vi "SHA-2_hash chunk_U64.vi"(0 "h in":u64[](array[numeric]), 1 "Chunk":u64[](array[numeric]), 12 "error in (no error)":errorcluster) -> (4 "h out":u64[](array[numeric]), 14 "error out":errorcluster)   [LabVIEW 2012, in "Encryption.lvlib"]
uses:
  Encryption.lvlib
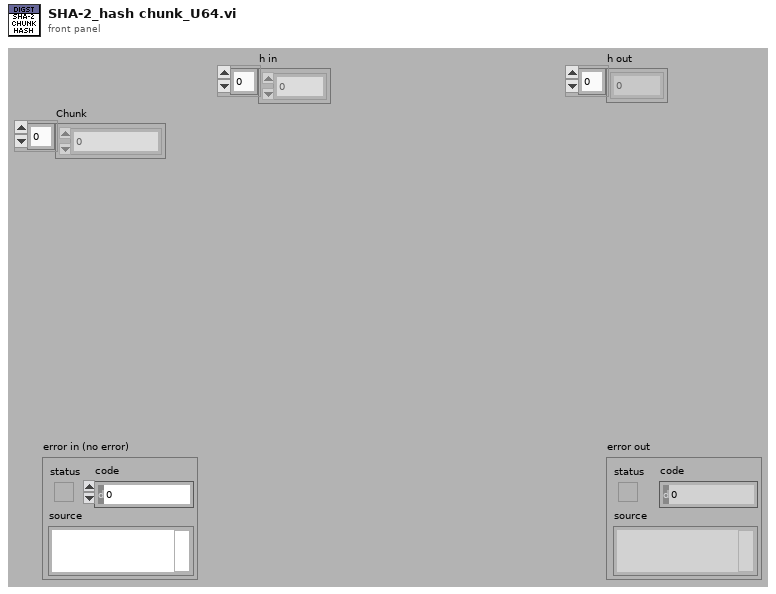
[diagram p1: front panel]
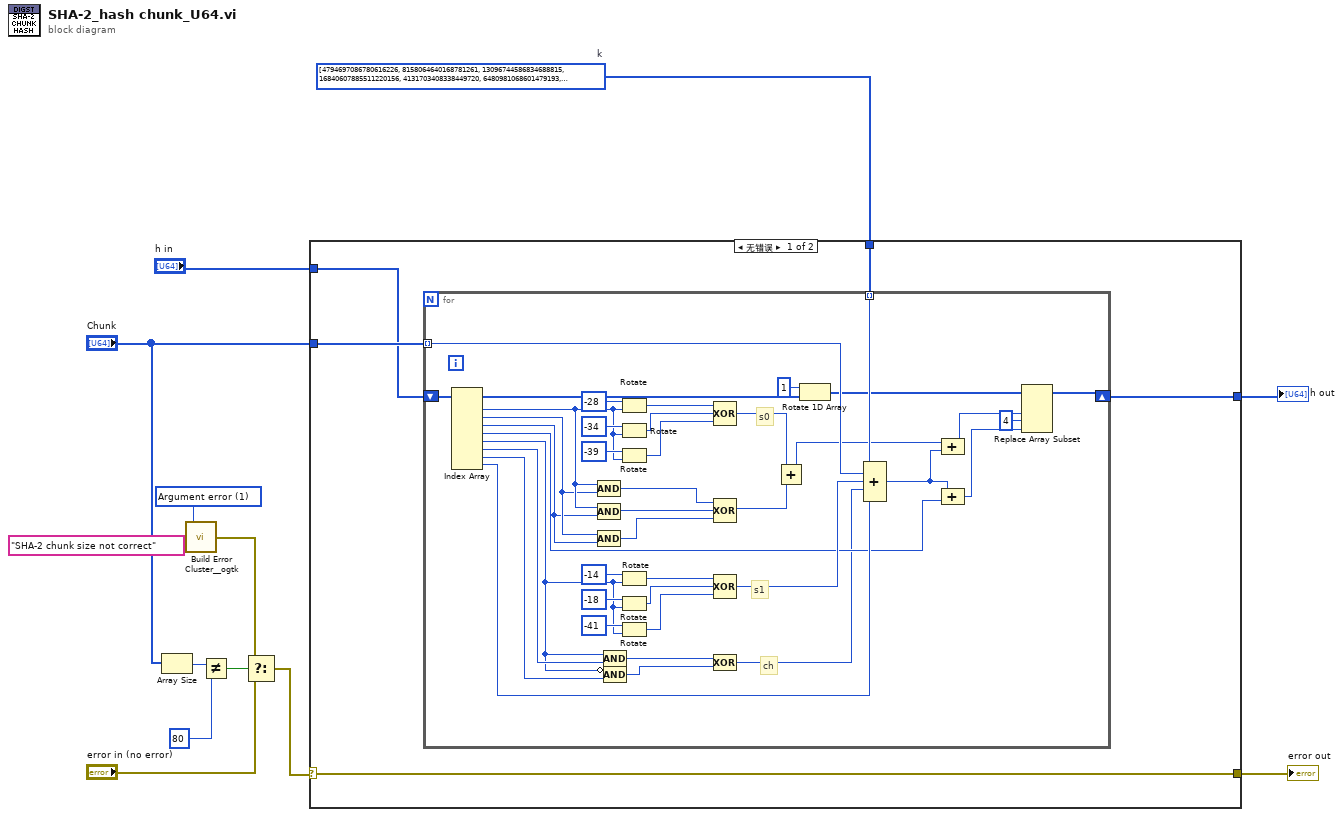
[diagram p0: block diagram]
diagram:
  w1 = u64[] [4794697086780616226, 8158064640168781261, 13096744586834688815, 16840607885511220156, 4131703408338449720, 6480981068601479193, 10538285296894168987, 12329834152419229976, 15566598209576043074, 1334009975649890238, 2608012711638119052, 6128411473006802146, 8268148722764581231, 9286055187155687089, 11230858885718282805, 13951009754708518548, 16472876342353939154, 17275323862435702243, 1135362057144423861, 2597628984639134821, 3308224258029322869, 5365058923640841347, 6679025012923562964, 8573033837759648693, 10970295158949994411, 12119686244451234320, 12683024718118986047, 13788192230050041572, 14330467153632333762, 15395433587784984357, 489312712824947311, 1452737877330783856, 2861767655752347644, 3322285676063803686, 5560940570517711597, 5996557281743188959, 7280758554555802590, 8532644243296465576, 9350256976987008742, 10552545826968843579, 11727347734174303076, 12113106623233404929, 14000437183269869457, 14369950271660146224, 15101387698204529176, 15463397548674623760, 17586052441742319658, 1182934255886127544, 1847814050463011016, 2177327727835720531, 2830643537854262169, 3796741975233480872, 4115178125766777443, 5681478168544905931, 6601373596472566643, 7507060721942968483, 8399075790359081724, 8693463985226723168, 9568029438360202098, 10144078919501101548, 10430055236837252648, 11840083180663258601, 13761210420658862357, 14299343276471374635, 14566680578165727644, 15097957966210449927, 16922976911328602910, 17689382322260857208, 500013540394364858, 748580250866718886, 1242879168328830382, 1977374033974150939, 2944078676154940804, 3659926193048069267, 4368137639120453308, 4836135668995329356, 5532061633213252278, 6448918945643986474, 6902733635092675308, 7801388544844847127]  # k
  w4 = 1 items=["No error", "Argument error", "Memory is full", "Out of zone", "End of file", "File already open", "Generic file I/O error", "File not found", "File permission error", "Disk is full", "Duplicate path", "Too many files open", "System feature not enabled", "Resource file not found", "Cannot add resource", "Resource not found", "Image not found", "Image memory error", "Pen does not exist", "Config type invalid", "Config token not found", "Config parse error", "Config memory error", "Bad external code format", "Bad external code offset", "External code not present", "Null window", "Destroy window error", "Null menu", "Print aborted", "Bad print record", "Print driver error", "Windows error during printing", "Memory error during printing", "Print dialog error", "Generic print error", "Invalid device refnum", "Device not found", "Device parameter error", "Device unit error", "Cannot open device", "Device call aborted", "Generic error", "Cancelled by user", "Object ID too low", "Object ID too high", "Object not in heap", "Unknown heap", "Unknown object (invalid DefProc)", "Unknown object (DefProc not in table)", "Message out of range", "Invalid (null) method", "Unknown message", "Manager call not supported", "Bad address", "Network operation in progress", "Network operation timed out", "Connection is busy", "Network attribute not supported", "Network error", "Address in use", "System out of memory", "Connection aborted", "Connection refused", "Not connected", "Already connected", "Connection closed", "Initialization error (interapplication manager)", "Bad occurrence", "Wait on unbound occurrence handler", "Occurrence queue overflow", "Datalog type conflict", "Unused", "Unrecognized type (interapplication manager)", "Memory corrupt", "Failed to make temporary DLL", "Old CIN version", "Drag socket not found", "Failed to load drop-object", "Failed to register OLE object", "Failed to release OLE object", "Format specifier type mismatch", "Unknown format specifier", "Too few format specifiers", "Too many format specifiers", "Scan failed", "Newer CIN version", "Error converting to variant", "Runtime menu error", "Password tampered", "Variant attribute not found", "Incompatible variant data type", "Event data is not available", "Event Store is not present", "Occurrence is not found", "Event Queue is not created", "Event info is not available", "Refnum passed is NULL", "Error retrieving Class GUID", "Error retrieving CoClass GUID", "Error retrieving TypeLib GUID.", "Bad built application magic bytes.", "Specific driver is different from the specific driver associated with the Logical Name.", "There is no session opened to the class driver.", "Max Error", "MAX - Error with config objects", "MAX - Error loading configuration", "MAX - Group not supported"]
  n1 = Array Size(array="Chunk") -> (size(s)=w12:i32)
  n2 = call <userlib>:"Build Error Cluster__ogtk.vi"("String to Prepend to source (\"\")"="SHA-2 chunk size not correct" ("String to Prepend to source (\"\")"), "code"=w4) -> ("error out"=w6:errorcluster)
  n3 = Not Equal?(x=w12, y=80) -> (x != y?=w10:bool)
  n4 = Select(t=w6, s=w10, f="error in (no error)") -> (s? t:f=w8:errorcluster)
  n5 = case shown="无错误" w8 {
    selector: w8 -> [w17 w59]
    tunnel: "Chunk" -> [w18 _]
    tunnel: [w17 w59] -> w7
    tunnel: [w16 _] -> w3
    tunnel: "h in" -> [w15 _]
    tunnel: w1 -> [w14 _]
    frame No Error {
      n6 = for {
        tunnel: w18 -> [w31] mode=indexing
        shift-right: [w26] -> w16
        shift-left: w15 -> [w29]
        tunnel: w14 -> [w32] mode=indexing
        # "ch"
        # "s1"
        # "s0"
        n7 = Index Array(array=w29) -> (element #1=w52:u64, element #2=w51:u64, element #3=w50:u64, element #4=w25:u64, element #5=w37:u64, element #6=w38:u64, element #7=w36:u64, element #8=w30:u64)  [unwired: 8 in]
        n8 = Compound Arithmetic op=AND(w52, w51) -> (w49:u64)
        n9 = Compound Arithmetic op=AND(w52, w50) -> (w48:u64)
        n10 = Compound Arithmetic op=AND(w51, w50) -> (w47:u64)
        n11 = Compound Arithmetic op=AND(w37, w38) -> (w35:u64)
        n12 = Compound Arithmetic op=AND(invert w37, w36) -> (w34:u64)
        n13 = Rotate(1:w52, 2:i8 -28 ("y")) -> (0:w57:u64)
        n14 = Rotate(1:w52, 2:i8 -34 ("y")) -> (0:w55:u64)
        n15 = Rotate(1:w52, 2:i8 -39 ("y")) -> (0:w53:u64)
        n16 = Rotate(1:w37, 2:i8 -14 ("y")) -> (0:w42:u64)
        n17 = Rotate(1:w37, 2:i8 -18 ("y")) -> (0:w44:u64)
        n18 = Rotate(1:w37, 2:i8 -41 ("y")) -> (0:w46:u64)
        n19 = Compound Arithmetic op=XOR(w57, w55, w53) -> (w40:u64)
        n20 = Compound Arithmetic op=XOR(w49, w48, w47) -> (w39:u64)
        n21 = Compound Arithmetic op=XOR(w42, w44, w46) -> (w33:u64)
        n22 = Compound Arithmetic op=XOR(w35, w34) -> (w20:u64)
        n23 = Add(x=w40, y=w39) -> (x+y=w22:u64)
        n24 = Rotate 1D Array(1:w29, 2:1 ("n")) -> (0:w27:u64[])
        n25 = Compound Arithmetic op=ADD(w32, w31, w33, w20, w30) -> (w19:u64)
        n26 = Compound Arithmetic op=ADD(w22, w19) -> (w21:u64)
        n27 = Compound Arithmetic op=ADD(w19, w25) -> (w24:u64)
        n28 = Replace Array Subset(array=w27, new element #1=w21, new element #2=w24, index #2=4 ("index")) -> (w26:u64[])  [unwired: 1 in]
      }
    }
    frame Error {
    }
  }
  "error out" <- w7
  "h out" <- w3
